vi "DAQ.Get Device Info.vi"(8 "error in (no error)":errorcluster, 11 "Instrument.DAQ":refnum<class "Instrument.DAQ.lvclass">) -> (0 "error out":errorcluster, 3 "Instrument.DAQ":refnum<class "Instrument.DAQ.lvclass">)   [LabVIEW 2019, in "Instrument.Lockin.lvlib" / "Instrument.DAQ.lvclass"]
uses:
  Instrument.DAQ.lvclass
  DAQmx/DAQmx.lvclass
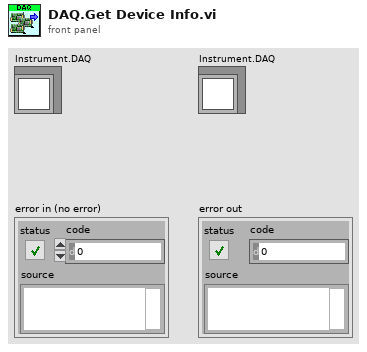
[diagram p1: front panel]
types:
  T1 = typedef "DAQmx.lvclass/DeviceInfo--Cluster.ctl" = cluster{"DeviceName":string, "DevIsSimulated":bool, "DeviceSerialNumber":u32, "ProductType":string, "ProductCategory":i32, "ProductNumber":u32, "ChassisNumber":u32, "SlotNumber":u32, "ChassisName":string, "ChassisSerialNumber":u32}
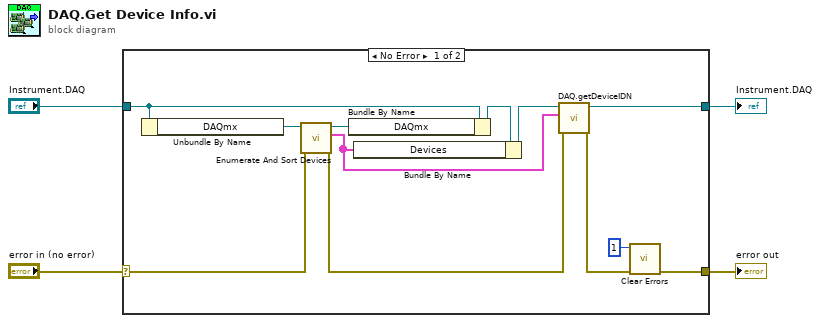
[diagram p0: block diagram]
diagram:
  n1 = case shown="No Error" "error in (no error)" {
    selector: "error in (no error)" -> [w6 w17]
    tunnel: "Instrument.DAQ" -> [w7 w18]
    tunnel: [w16 w18] -> w2
    tunnel: [w14 w17] -> w1
    frame No Error {
      n2 = Unbundle By Name(w7) -> ("DAQmx"=w12:refnum<class "DAQmx.lvclass">)
      n3 = call "Enumerate And Sort Devices.vi"("error in (no error)"=w6, "DAQmx in"=w12) -> ("error out"=w11:errorcluster, "Devices (sorted)"=w5:T1[], "DAQmx out"=w10:refnum<class "DAQmx.lvclass">)  [unwired: 7 in]
      n4 = Bundle By Name(cluster=w7, "DAQmx"=w10) -> (w9:refnum<class "Instrument.DAQ.lvclass">)
      n5 = Bundle By Name(cluster=w9, "Devices"=w5) -> (w8:refnum<class "Instrument.DAQ.lvclass">)
      n6 = call "DAQ.getDeviceIDN.vi"("error in (no error)"=w11, "Devices"=w5, "Instrument.DAQ"=w8) -> ("error out"=w15:errorcluster, "Instrument.DAQ out"=w16:refnum<class "Instrument.DAQ.lvclass">)  [unwired: 7 in]
      n7 = call <vilib>:"Clear Errors.vi"("error in (no error)"=w15, "specific error code to clear (0: all)"=1) -> ("error out"=w14:errorcluster)  [unwired: 4 in, 1 out]
    }
    frame Error {
    }
  }
  "Instrument.DAQ" <- w2
  "error out" <- w1
